vi "NATS Client start.vi"(6 "timeout ms (5)":i32=5, 8 "error in":errorcluster {"code" format="Error %.0f"}, 9 "bytes to read (1024)":i32=1024, 10 "port (4222)":u16=4222, 11 "address":string="localhost") -> (0 "error out":errorcluster {"code" format="Error %.0f"}, 3 "NATS Client out":refnum<class "NATS Client.lvclass">)   [LabVIEW 2024, in "NATS Client.lvlib" / "NATS Client.lvclass"]
uses:
  NATS Client.lvclass
  subscription queue.ctl
  subscription actions.ctl
  NATS Subscription/NATS Subscription.lvclass
  NATS Client.lvclass/NATS Client.ctl
  set async stop notifier.vi
  set subscriptions queue.vi
  set async vi.vi
  set nats connection.vi
  VIs/subVIs/Set Timeout.vi
  VIs/subVIs/Validate CONNECT.vi
  VIs/NATS PING.vi
  <vilib>/Utility/error.llb/Trim Whitespace.vi
  VIs/subVIs/Check for Authorization.vi
  VIs/subVIs/Add Version and Language JSON Entries.vi
  <vilib>/Utility/error.llb/Trim Whitespace One-Sided.vi
  VIs/subVIs/Package Version Constant.vi
  client.vi
  VIs/NATS READ.vi
  NATS Core.lvlib
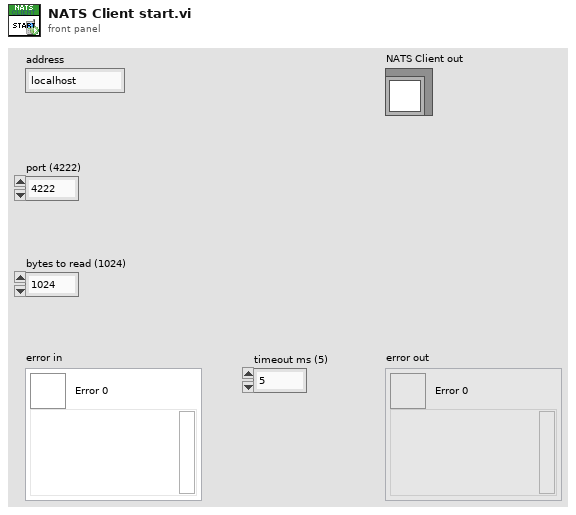
[diagram p1: front panel]
types:
  T1 = typedef "NATS Client.lvlib/NATS Client.lvclass/subscription queue.ctl" = cluster{"action":T2, "subscription":refnum<class "NATS Subscription.lvclass">}
  T2 = typedef "NATS Client.lvlib/NATS Client.lvclass/subscription actions.ctl" = enum16{"sub", "unsub"}
  T3 = typedef "NATS Core.lvlib/nats connection.ctl" = cluster{"connection ID":refnum<k5>, "server INFO":string, "timeout ms":i32, "verbose?":bool, "server headers?":bool, "client headers?":bool}
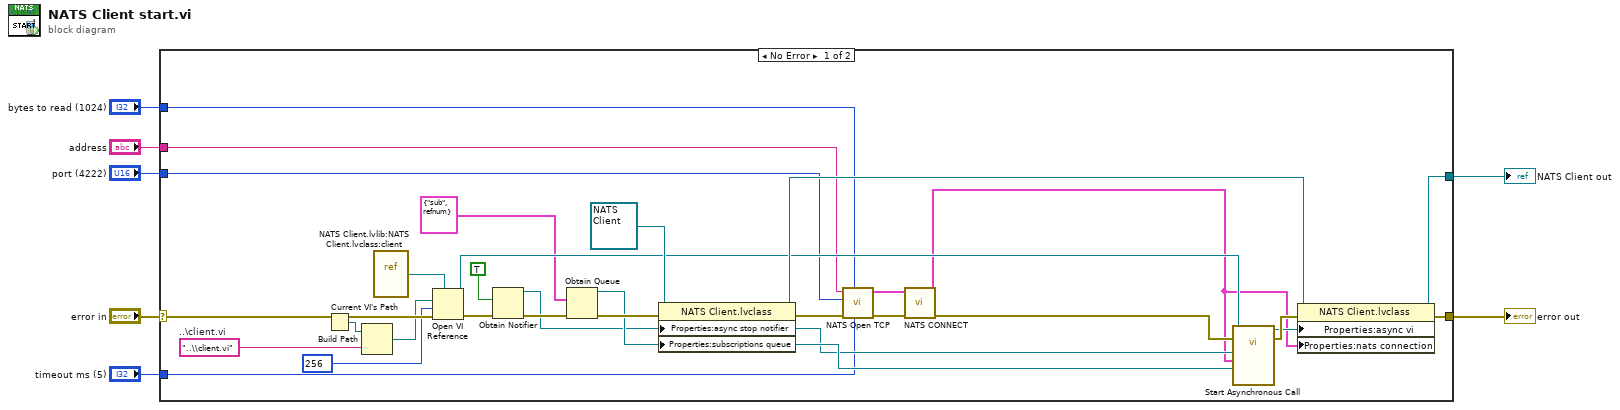
[diagram p0: block diagram]
diagram:
  n1 = case shown="No Error" "error in" {
    selector: "error in" -> [w36 w37]
    tunnel: [w33 w37] -> w6
    tunnel: [w20 _] -> w5
    tunnel: "address" -> [w12 _]
    tunnel: "bytes to read (1024)" -> [w10 _]
    tunnel: "timeout ms (5)" -> [w9 _]
    tunnel: "port (4222)" -> [w8 _]
    frame No Error {
      w24 = "..\\client.vi"  # ..\client.vi
      n2 = Current VI's Path() -> (path=w26:path)
      n3 = Build Path(base path=w26, name or relative path=w24) -> (appended path=w23:path)
      n4 = vi-ref "NATS Client.lvlib:NATS Client.lvclass:client.vi"() -> (w27:refnum<vi>)
      n5 = Open VI Reference(type specifier VI Refnum (for type only)=w27, vi path=w23, options=256, error in (no error)=w36) -> (vi reference=w19:refnum<vi>, error out=w35:errorcluster)  [unwired: 2 in]
      n6 = Obtain Notifier(notification data type=TRUE ("create if not found?"), error in (no error)=w35) -> (notifier out=w14:refnum<notifier>, error out=w32:errorcluster)  [unwired: 2 in, 1 out]
      n7 = Obtain Queue(element data type=T1 {"action"=enum."sub", "subscription"=refnum} ("subscription queue"), error in (no error)=w32) -> (queue out=w15:refnum<queue>, error out=w34:errorcluster)  [unwired: 3 in, 1 out]
      n8 = property class="NATS Client.lvclass"(reference=refnum<class "NATS Client.lvclass"> refnum ("NATS Client out"), error in=w34, "Properties:async stop notifier"=w14, "Properties:subscriptions queue"=w15) -> (reference out=w21:refnum<class "NATS Client.lvclass">, error out=w30:errorcluster)
      n9 = call "NATS Open TCP.vi"("timeout ms (5000)"=w9, "bytes to read (1024)"=w10, "error in"=w30, "port (4222)"=w8, "address"=w12) -> ("error out"=w31:errorcluster, "nats connection"=w16:T3)  [unwired: 3 in, 2 out]
      n10 = call "NATS CONNECT.vi"("error in"=w31, "nats connection in"=w16) -> ("error out"=w28:errorcluster, "nats connection out"=w11:T3)  [unwired: 7 in, 1 out]
      n11 = call-by-ref "Start Asynchronous Call"(reference=w19, error in=w28, "subscriptions queue"=w15, "nats connection"=w11, "async stop notifier"=w14) -> (reference out=w17:refnum<vi>, error out=w29:errorcluster)  [unwired: 8 in, 1 out]
      n12 = property class="NATS Client.lvclass"(reference=w21, error in=w29, "Properties:async vi"=w17, "Properties:nats connection"=w11) -> (reference out=w20:refnum<class "NATS Client.lvclass">, error out=w33:errorcluster)
    }
    frame Error {
    }
  }
  "error out" <- w6
  "NATS Client out" <- w5
